vi "PE Get Grating Name.vi"(8 "error in (no error)":errorcluster, 10 "gratingIndex":i32, 11 "peHandle":u32) -> (0 "error out":errorcluster, 3 "name":string)   [LabVIEW 2017, in "PE_Filter_SDK.lvlib"]
doc: "PEFILTERSDK_API PE_STATUS PE_GetGratingName(CPE_HANDLE peHandle, int gratingIndex, char* name, int size);"
uses:
  PE_Filter_SDK.lvlib
  PE_Filter_SDK.dll
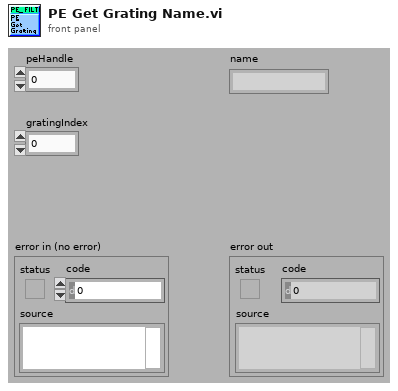
[diagram p1: front panel]
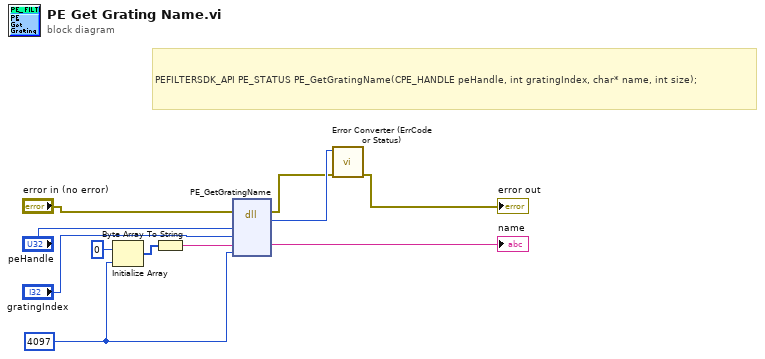
[diagram p0: block diagram]
diagram:
  w7 = 4097 ("size")
  # "PEFILTERSDK_API PE_STATUS PE_GetGratingName(CPE_HANDLE peHandle, int gratingIndex, char* name, int size);"
  n1 = Initialize Array(u8 0 ("element"), w7) -> (w9:u8[])
  n2 = Byte Array To String(unsigned byte array=w9) -> (string=w8:string)
  n3 = dll-call lib="PE_Filter_SDK.*" fn="PE_GetGratingName"(error in="error in (no error)", "peHandle"="peHandle", "gratingIndex"="gratingIndex", "name"=w8, "size"=w7) -> (error out=w2:errorcluster, w3:u32, "name"=→"name":string)  [unwired: 5 in, 1 out]
  n4 = call "Error Converter (ErrCode or Status).vi"("error in (no error)"=w2, "error code"=w3) -> ("error out"=→"error out":errorcluster)  [unwired: 9 in]
